vi "Init.vi"(8 "Creator Attributes":T1, 9 "Self Attributes":T1, 10 "Register":refnum<event-registration>) -> (3 "Base Actor out":refnum<class "Base Actor.lvclass">)   [LabVIEW 2020, in "jettl.lvlib" / "Actor.lvlib" / "Base Actor.lvclass"]
uses:
  Base Actor.lvclass
  Msg/Msg.lvclass
  Implemented Msgs.ctl
  Actor.lvlib
  Attributes.ctl
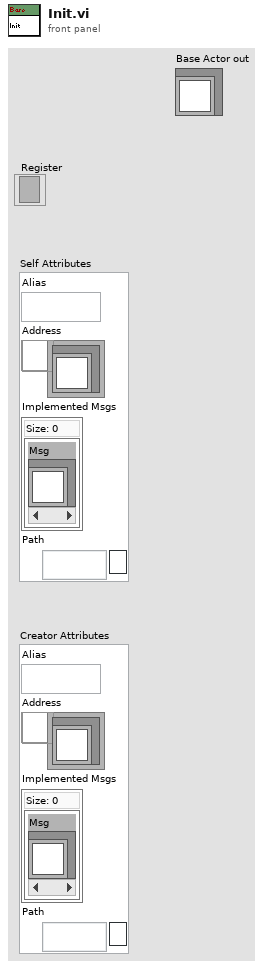
[diagram p1: front panel]
types:
  T1 = typedef "jettl.lvlib/Actor.lvlib/Attributes.ctl" = cluster{"Alias":string, "Address":refnum<user-event>, "Implemented Msgs":T2, "Path":path}
  T2 = typedef "jettl.lvlib/Actor.lvlib/Implemented Msgs.ctl" = set{refnum<class "Msg.lvclass">}
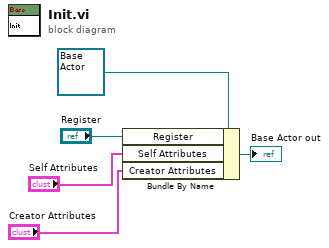
[diagram p0: block diagram]
diagram:
  n1 = Bundle By Name(cluster=refnum<class "Base Actor.lvclass"> refnum ("jettl Event Actor out"), "Register"="Register", "Self Attributes"="Self Attributes", "Creator Attributes"="Creator Attributes") -> (→"Base Actor out":refnum<class "Base Actor.lvclass">)
